vi "Logger.Variant.GetDMCConfig.vi"(8 "error in (no error)":errorcluster) -> (0 "error out":errorcluster, 2 "DMCconfig":i32[](array[numeric]))   [LabVIEW 2016]
uses:
  Global/ApplicationGlobal.vi
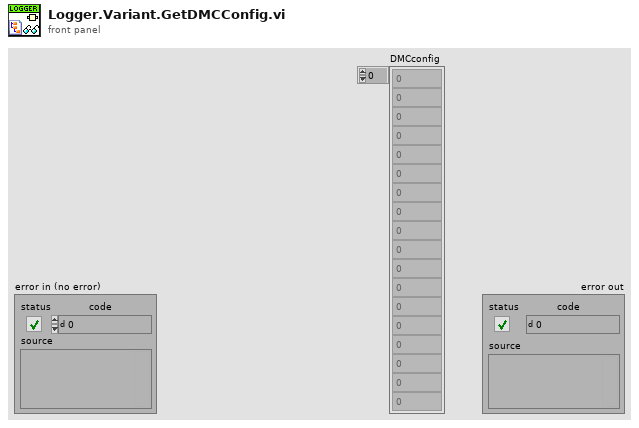
[diagram p1: front panel]
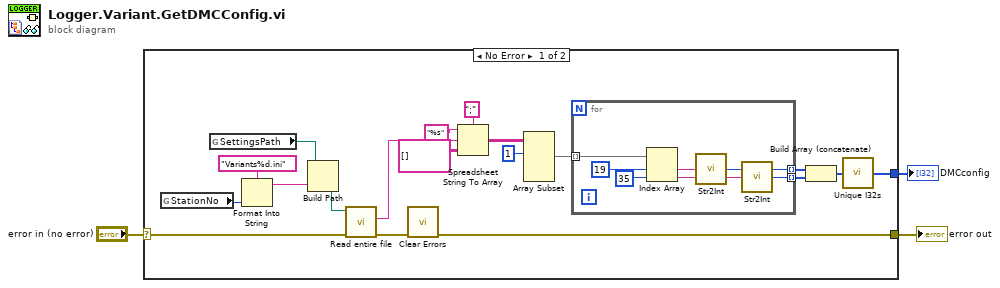
[diagram p0: block diagram]
diagram:
  n1 = case shown="No Error" "error in (no error)" {
    selector: "error in (no error)" -> [w22 w30]
    tunnel: [w14 w30] -> w2
    tunnel: [w8 _] -> w1
    frame No Error {
      n2 = global read "ApplicationGlobal.vi" "StationNo"() -> (w4:i32)
      n3 = global read "ApplicationGlobal.vi" "SettingsPath"() -> (w7:path)
      n4 = Format Into String(format string="Variants%d.ini", w4) -> (resulting string=w6:string)  [unwired: 2 in, 1 out]
      n5 = Build Path(base path=w7, name or relative path=w6) -> (appended path=w21:path)
      n6 = call "Read entire file.vi"("error in"=w22, "file"=w21) -> ("error out"=w15:errorcluster, "contents"=w20:string)  [unwired: 4 in]
      n7 = call <vilib>:"Clear Errors.vi"("error in (no error)"=w15) -> ("error out"=w14:errorcluster)  [unwired: 5 in, 1 out]
      n8 = Spreadsheet String To Array(delimiter (Tab)=";", format string="%s", spreadsheet string=w20, array type (2D Dbl)=string[][] []) -> (array=w13:string[][])
      n9 = Array Subset(array=w13, index (row)=1 ("index")) -> (w12:string[][])  [unwired: 3 in]
      n10 = for {
        tunnel: w12 -> [w25] mode=indexing
        tunnel: [w24] -> w11 mode=indexing
        tunnel: [w23] -> w10 mode=indexing
        n11 = Index Array(array=w25, index #1=19 ("index"), index #2=35 ("index")) -> (element #1=w27:string, element #2=w26:string)
        n12 = call "Str2Int.vi"("string"=w27) -> ("Numeric"=w24:i32)
        n13 = call "Str2Int.vi"("string"=w26) -> ("Numeric"=w23:i32)
      }
      n14 = Build Array (concatenate)(w11, w10) -> (w9:i32[])
      n15 = call "Unique I32s.vi"("values in"=w9) -> ("unique values"=w8:i32[])
    }
    frame Error {
    }
  }
  "error out" <- w2
  "DMCconfig" <- w1
